vi "Save_Mes_en.vi"(5 "error in (no error)":errorcluster caption="错误输入（无错误）") -> (15 "元素":bool, 16 "value":dbl caption="值", 19 "error out":errorcluster caption="错误输出")   [LabVIEW 2018]
uses:
  Global.vi
  <vilib>/Utility/config.llb/Read Key (Double).vi
  <vilib>/Utility/config.llb/NI_LVConfig.lvlib
panel:
  out "布尔数组":bool[](array[boolean])
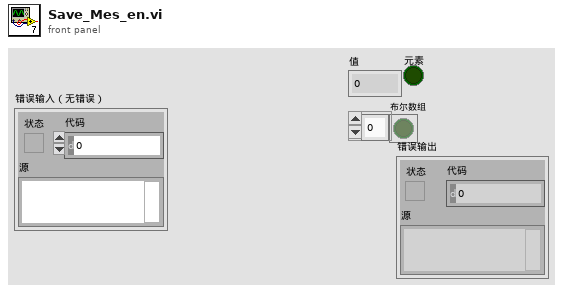
[diagram p1: front panel]
types:
  T1 = typedef "NI_LVConfig.lvlib/Config Data RefNum.ctl" = refnum<k1>
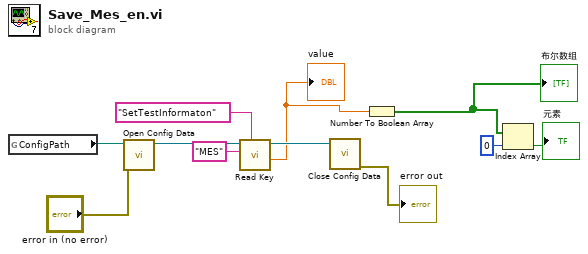
[diagram p0: block diagram]
diagram:
  n1 = global read "Global.vi" "ConfigPath"() -> (w11:path)
  n2 = call <vilib>:"Open Config Data.vi"("error in (no error)"="error in (no error)", "configuration file path"=w11) -> ("refnum"=w10:T1)  [unwired: 7 in, 2 out]
  n3 = call-poly <vilib>:"Read Key.vi"("section"="SetTestInformaton", "key"="MES", "refnum"=w10) -> ("value"=w6:dbl, "refnum out"=w7:T1)  [unwired: 5 in, 2 out]
  "value" <- w6
  n4 = call <vilib>:"Close Config Data.vi"("refnum"=w7) -> ("error out"=→"error out":errorcluster)  [unwired: 9 in, 1 out]
  n5 = Number To Boolean Array(number=w6) -> (Boolean array=w5:bool[])
  "布尔数组" <- w5
  n6 = Index Array(array=w5, index=0 ("索引")) -> (element=→"元素":bool)
